vi "Write Force Setpoint.vi"(10 "Force Setpoint":T1 min=-888.0 max=888.0 format="%.2f", 11 "SystemController in":refnum<class "SystemController.lvclass">) -> (3 "SystemController out":refnum<class "SystemController.lvclass">)   [LabVIEW 2013, in "SystemController.lvclass"]
uses:
  SystemController.lvclass
  Typedefs/ForceSetpoint.ctl
  SystemController.lvclass/SystemController.ctl
  Typedefs/FAMTTypedefs.lvlib
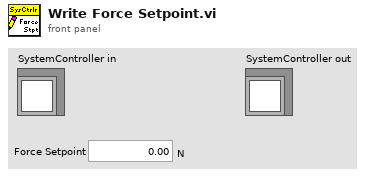
[diagram p1: front panel]
types:
  T1 = typedef "FAMTTypedefs.lvlib/ForceSetpoint.ctl" = dbl[unit]
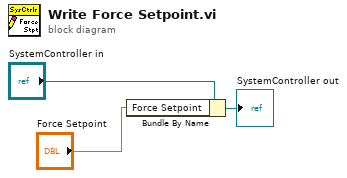
[diagram p0: block diagram]
diagram:
  n1 = Bundle By Name(cluster="SystemController in", "Force Setpoint"="Force Setpoint") -> (→"SystemController out":refnum<class "SystemController.lvclass">)
